vi "write_error_type.vi"(10 "error_type":T1, 11 "Error in":refnum<class "Error.lvclass">) -> (3 "Error out":refnum<class "Error.lvclass">)   [LabVIEW 2023, in "Error Handling Interface.lvlib" / "Error.lvclass"]
uses:
  Error.lvclass
  error_type.ctl
  Error.lvclass/Error.ctl
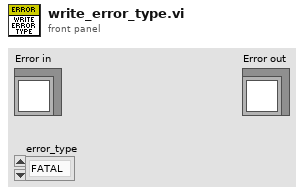
[diagram p1: front panel]
types:
  T1 = typedef "Error Handling Interface.lvlib/Error.lvclass/error_type.ctl" = enum16{"FATAL", "ERROR", "WARNING", "INFO", "DEBUG", "TRACE"}
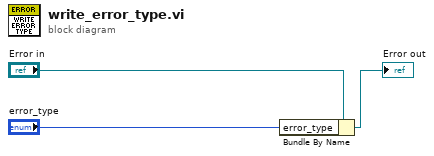
[diagram p0: block diagram]
diagram:
  n1 = Bundle By Name(cluster="Error in", "error_type"="error_type") -> (→"Error out":refnum<class "Error.lvclass">)
